vi "dotNET Crypto Demonstrator.vi"() -> ()   [LabVIEW 2021]
uses:
  Asymmetric Encryption/RSA/RSAEncryptionPadding.ctl
  Asymmetric Encryption/RSA/RSASignaturePadding.ctl
  Asymmetric Encryption/RSA/HashingAlgorithm.ctl
  Random Number Generation/dotNET Crypto RNG.lvlib
  Key Derivation/dotNET Crypto Key Derivation.lvlib
  Hashing/dotNET Crypto Hashing.lvlib
  Utility/dotNET Crypto Utility.lvlib
  Key Management/dotNET Crypto Key Management.lvlib
  Symmetric Encryption/dotNET Crypto Symmetric Encryption.lvlib
  System.Core
  Asymmetric Encryption/dotNET Crypto Asymmetric Encryption.lvlib
panel:
  in  "Tab Control":T1(tab)
  out "Random Data (hex string)":string
  in  "Gen RNG":bool
  out "Random Data (byte)":u8[](array[numeric])
  in  "# bytes":i32=32
  in  "Hashed Password (existing salt)":string
  out "Match?":bool
  in  "PBKDF2 Verify":bool
  in  "Salt":string
  in  "Hashed Password (random salt)":string
  in  "PBKDF2 Hash":bool
  in  "Password":string
  in  "HashingAlgorithm (SHA512)":T2=enum."SHA512"
  in  "Key length (64 bytes)":i32=64
  in  "saltSize (16 bytes)":i32=16
  in  "iterations (210000)":i32=210000
  in  "SHA512":bool
  in  "SHA384":bool
  in  "SHA256":bool
  in  "SHA1":bool
  in  "MD5":bool
  in  "Hash Out (hex string)":string
  in  "Data In":string
  in  "Hash Format":enum16{"ASCII", "Hex String"}(ring)
  in  "Cipher Block Mode":enum16{"ECB", "CBC"}(ring)=enum."CBC"
  in  "Initialisation Vector (hex string)":string
  in  "Create AES Key":bool
  in  "Key Size":enum16{"128 bit", "192 bit", "256 bit"}(ring)=enum."256 bit"
  in  "AES Key (hex string)":string
  in  "AES Encrypted Data":string
  in  "AES Raw Data":string
  in  "AES Encrypt":bool
  in  "AES Decrypt":bool
  in  "AES Encrypted Format":enum16{"ASCII", "Hex String"}(ring)=enum."Hex String"
  in  "AES Raw Format":enum16{"ASCII", "Hex String"}(ring)
  in  "Padding Mode":i32(ring)=3 items=["None"=1, "PKCS7"=2, "Zeros"=3, "ANSIX923"=4, "ISO10126"=5]
  in  "RSA Raw Format":enum16{"ASCII", "Hex String"}(ring)
  in  "RSA Encrypted Format":enum16{"ASCII", "Hex String"}(ring)=enum."Hex String"
  in  "RSA Decrypt":bool
  in  "RSA Encrypt":bool
  in  "Public Key (hex string)":string
  in  "Private Key (hex string)":string
  in  "Create RSA KeyPair":bool
  in  "RSA Encrypted Data":string
  in  "RSA Raw Data":string
  in  "keySize (2048 bit)":i32=2048
  in  "Padding Mode":T3=enum."OaepSHA512"
  out "Verified?":bool
  in  "RSASign Data Format":enum16{"ASCII", "Hex String"}(ring)
  in  "RSA Verify Data":bool
  in  "RSA Sign Data":bool
  in  "Signing Public Key (hex string)":string
  in  "Signing Private Key (hex string)":string
  in  "Create RSA Signing KeyPair":bool
  in  "Signature (hex string)":string
  in  "Data To Sign / Verify":string
  in  "keySize (2048 bit)":i32=2048
  in  "Signature Padding":T4
  in  "HashingAlgorithm":T2=enum."SHA512"
  in  "Key Length (bytes)":i32=64
  in  "Hash Algorithm":enum16{"HMACSHA256", "HMACSHA512"}(ring)
  in  "Generate Signature":bool
  in  "HMAC Signature (hex string)":string
  in  "HMAC Data Format":enum16{"ASCII", "Hex String"}(ring)
  in  "HMAC Data":string
  in  "HMAC Key (hex string)":string
  in  "Create HMAC Key":bool
  # ".NET Cryptography Library Playground"
  # "Generate random bytes of data using a cryptographically secure algorithm."
  # "Generates a fixed length key from an input password - can be used for key derivation or password hashing."
  # "Step 1: Generate a computationally intensive hash from the provided password."
  # "Step 2: Verify the password against the hash (reusing the previous salt above)"
  # "Generates a hash from the input data."
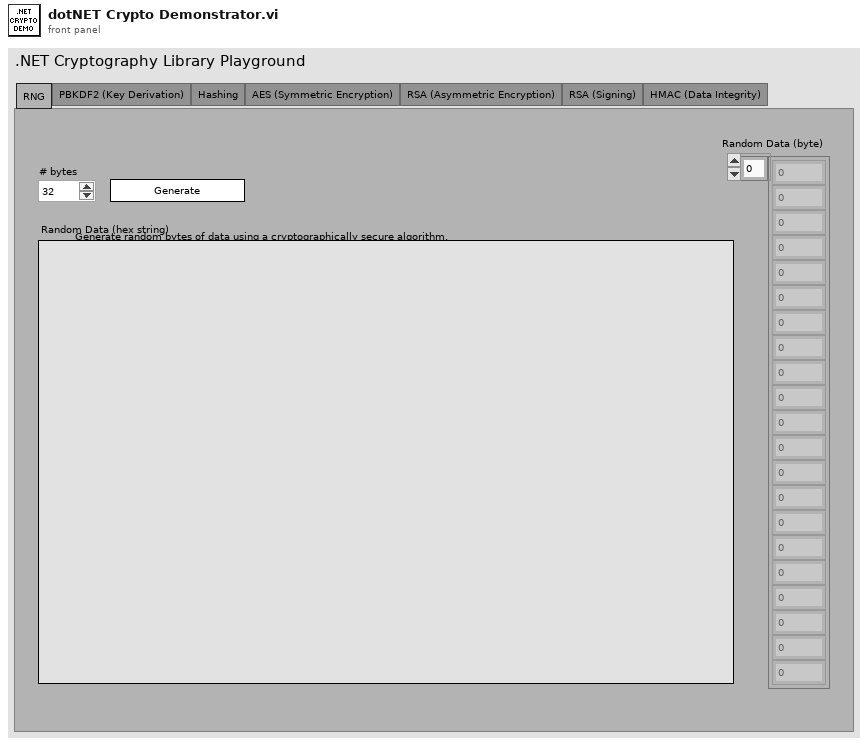
[diagram p1: front panel]
types:
  T1 = enum32{"RNG", "PBKDF2 (Key Derivation)", "Hashing", "AES (Symmetric Encryption)", "RSA (Asymmetric Encryption)", "RSA (Signing)", "HMAC (Data Integrity)"}
  T2 = typedef "dotNET Crypto Utility.lvlib/HashingAlgorithm.ctl" = enum16{"MD5", "SHA1", "SHA256", "SHA384", "SHA512"}
  T3 = typedef "dotNET Crypto Asymmetric Encryption.lvlib/RSAEncryptionPadding.ctl" = enum16{"OaepSHA1", "OaepSHA256", "OaepSHA384", "OaepSHA512", "Pkcs1"}
  T4 = typedef "dotNET Crypto Asymmetric Encryption.lvlib/RSASignaturePadding.ctl" = enum16{"Pkcs1", "Pss"}
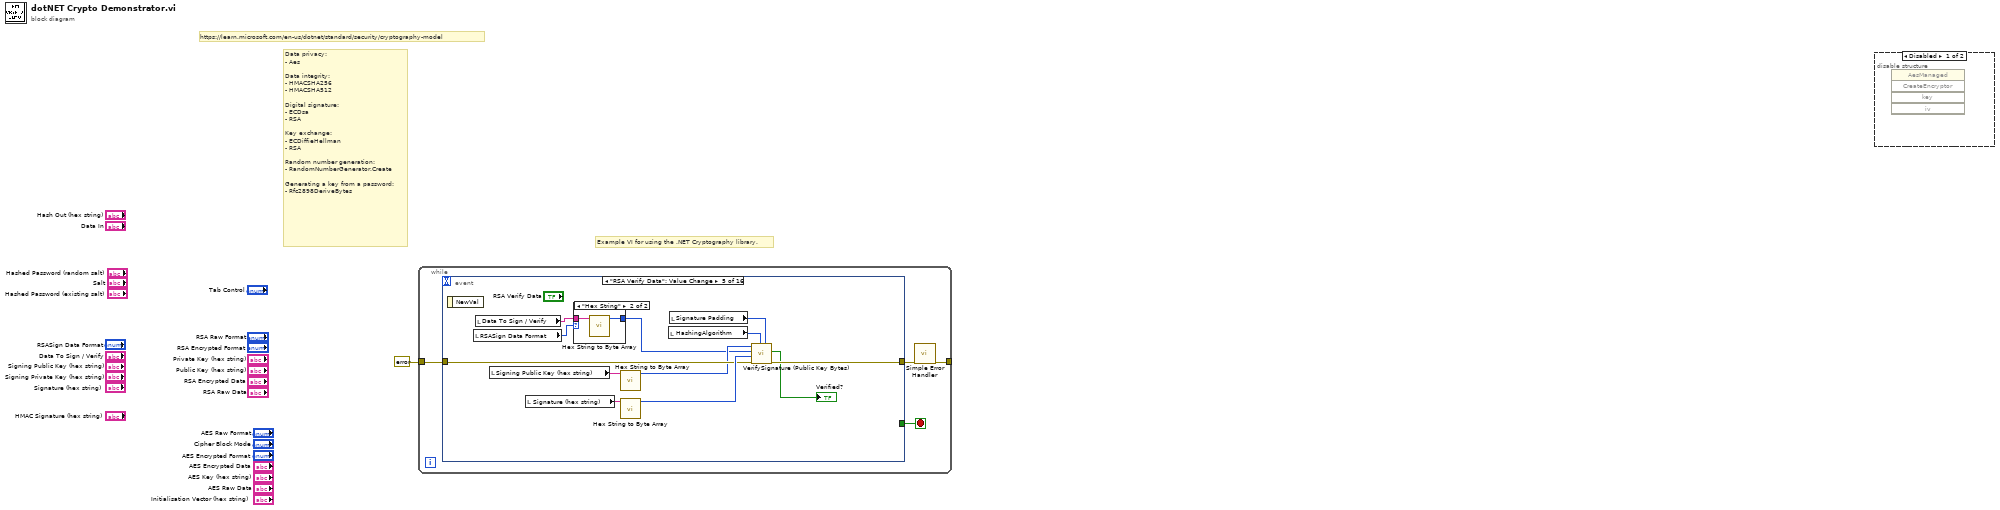
[diagram p0: block diagram]
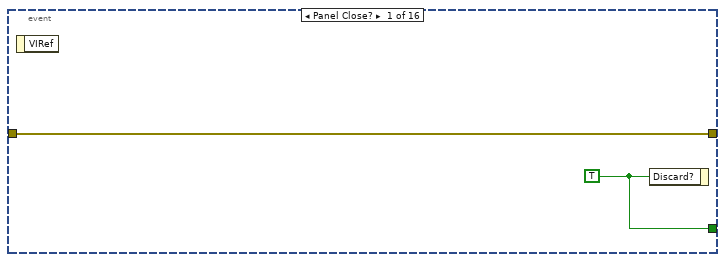
[diagram p2: hidden frame]
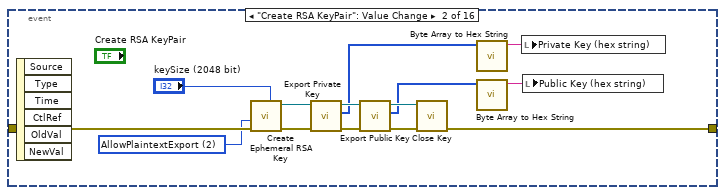
[diagram p3: hidden frame]
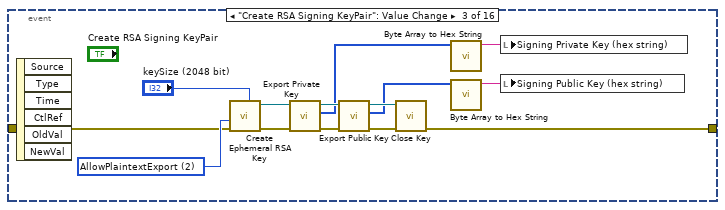
[diagram p4: hidden frame]
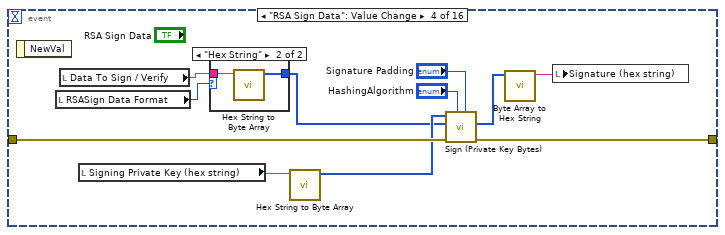
[diagram p5: hidden frame]
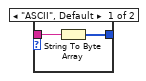
[diagram p6: hidden frame]
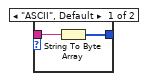
[diagram p7: hidden frame]
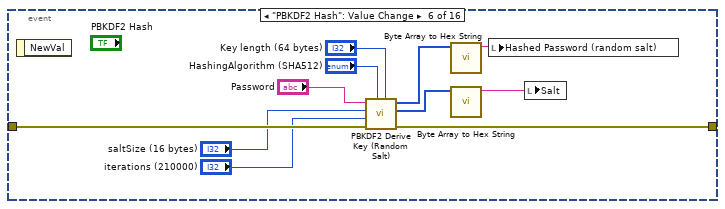
[diagram p8: hidden frame]
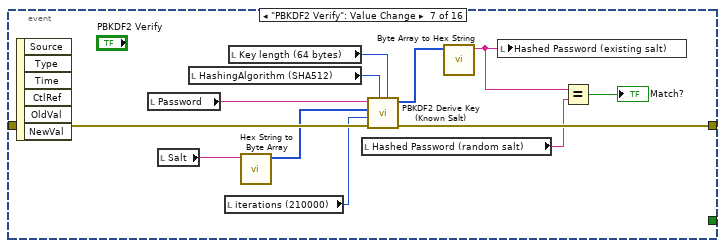
[diagram p9: hidden frame]
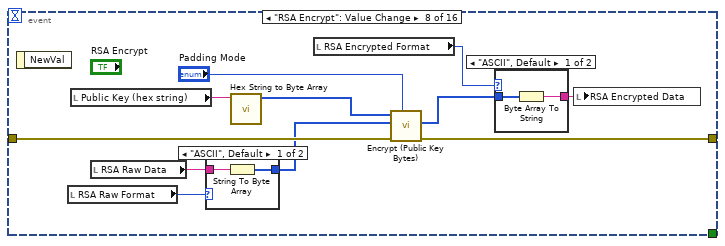
[diagram p10: hidden frame]
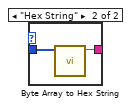
[diagram p11: hidden frame]
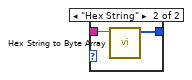
[diagram p12: hidden frame]
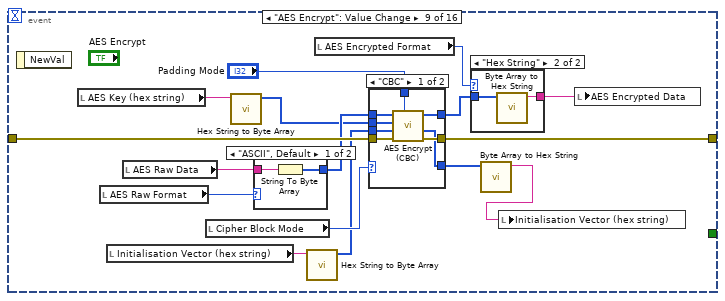
[diagram p13: hidden frame]
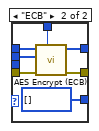
[diagram p14: hidden frame]
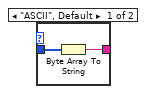
[diagram p15: hidden frame]
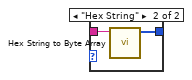
[diagram p16: hidden frame]
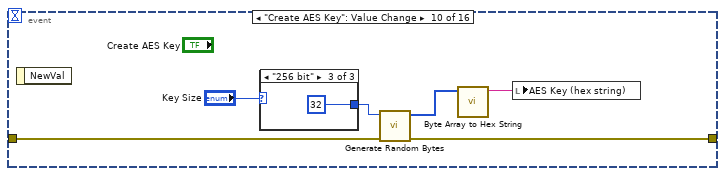
[diagram p17: hidden frame]
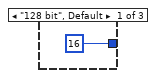
[diagram p18: hidden frame]
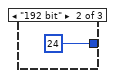
[diagram p19: hidden frame]
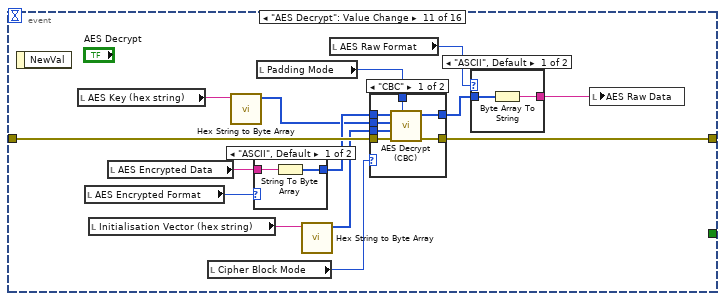
[diagram p20: hidden frame]
diagram:
  # "Example VI for using the .NET Cryptography library."
  # "https://learn.microsoft.com/en-us/dotnet/standard/security/cryptography-model"
  # "Data privacy:\n- Aes\n\nData integrity:\n- HMACSHA256\n- HMACSHA512\n\nDigital signature:\n- ECDsa\n- RSA\n\nKey exchange:\n- ECDiffieHellman\n- RSA\n\nRandom number generation:\n- RandomNumberGenerator.Create\n\nGenerating a key from a password:\n- Rfc2898DeriveBytes"
  n1 = while {
    tunnel: [w2] -> _
    tunnel: errorcluster {"status"=FALSE, "code"=0, "source"=""} ("error out") -> [w3]
    stop <- w5 stop-if-true
    n2 = event shown="[4] \"RSA Verify Data\": Value Change" {
      selector: _ -> [_ _ _ _ _ _ _ _ _ _ _ _ _ _ _ _]
      dyn-events: _ -> [_ _ _ _ _ _ _ _ _ _ _ _ _ _ _ _]
      timeout: _ -> [_ _ _ _ _ _ _ _ _ _ _ _ _ _ _ _]
      tunnel: [w7 _ _ _ _ _ _ _ _ _ _ _ _ _ _ _] -> w5
      tunnel: [w6 w17 w25 w46 w62 w76 w89 w93 w123 w150 w169 w195 w214 w223 w261 w280] -> w4
      tunnel: w3 -> [w6 w21 w26 w39 w53 w77 w88 w92 w124 w153 w170 w194 w213 w224 w262 w281]
      event Panel Close? {
        w7 = TRUE ("Discard?")
        n3 = event-data() -> ()  [unwired: 1 in, 1 out]
        n4 = event-data("Discard?"=w7) -> ()  [unwired: 1 in, 1 out]
      }
      event "Create RSA KeyPair": Value Change {
        w16 = 2 items=["None"=0, "AllowExport"=1, "AllowPlaintextExport"=2, "AllowArchiving"=4, "AllowPlaintextArchiving"=8] ("Export Policy (allow export)")
        n5 = event-data() -> ()  [unwired: 1 in, 6 out]
        n6 = call "Create Ephemeral RSA Key.vi"("Key Length (2048)"="keySize (2048 bit)", "error in (no error)"=w21, "Export Policy (allow export)"=w16) -> ("error out"=w15:errorcluster, "CngKey out"=w10:refnum<k24>)  [unwired: 7 in]
        n7 = call "Export Private Key.vi"("error in (no error)"=w15, "CngKey ref in"=w10) -> ("error out"=w14:errorcluster, "Private Key"=w9:u8[], "CngKey ref out"=w11:refnum<k24>)  [unwired: 7 in]
        n8 = call "Export Public Key.vi"("error in (no error)"=w14, "CngKey ref in"=w11) -> ("error out"=w13:errorcluster, "Public Key"=w8:u8[], "CngKey ref out"=w12:refnum<k24>)  [unwired: 7 in]
        n9 = call "Close Key.vi"("error in (no error)"=w13, "CngKey in"=w12) -> ("error out"=w17:errorcluster)  [unwired: 9 in]
        n10 = call "Byte Array to Hex String.vi"("Byte Array"=w9) -> ("Hex String"=w20:string)  [unwired: 10 in]
        n11 = call "Byte Array to Hex String.vi"("Byte Array"=w8) -> ("Hex String"=w19:string)  [unwired: 10 in]
        n12 = local write "Private Key (hex string)"(w20) -> ()
        n13 = local write "Public Key (hex string)"(w19) -> ()
      }
      event "Create RSA Signing KeyPair": Value Change {
        w33 = 2 items=["None"=0, "AllowExport"=1, "AllowPlaintextExport"=2, "AllowArchiving"=4, "AllowPlaintextArchiving"=8] ("Export Policy (allow export)")
        n14 = event-data() -> ()  [unwired: 1 in, 6 out]
        n15 = call "Create Ephemeral RSA Key.vi"("Key Length (2048)"="keySize (2048 bit)", "error in (no error)"=w26, "Export Policy (allow export)"=w33) -> ("error out"=w32:errorcluster, "CngKey out"=w27:refnum<k24>)  [unwired: 7 in]
        n16 = call "Export Private Key.vi"("error in (no error)"=w32, "CngKey ref in"=w27) -> ("error out"=w31:errorcluster, "Private Key"=w23:u8[], "CngKey ref out"=w28:refnum<k24>)  [unwired: 7 in]
        n17 = call "Export Public Key.vi"("error in (no error)"=w31, "CngKey ref in"=w28) -> ("error out"=w30:errorcluster, "Public Key"=w22:u8[], "CngKey ref out"=w29:refnum<k24>)  [unwired: 7 in]
        n18 = call "Close Key.vi"("error in (no error)"=w30, "CngKey in"=w29) -> ("error out"=w25:errorcluster)  [unwired: 9 in]
        n19 = call "Byte Array to Hex String.vi"("Byte Array"=w23) -> ("Hex String"=w35:string)  [unwired: 10 in]
        n20 = call "Byte Array to Hex String.vi"("Byte Array"=w22) -> ("Hex String"=w34:string)  [unwired: 10 in]
        n21 = local write "Signing Private Key (hex string)"(w35) -> ()
        n22 = local write "Signing Public Key (hex string)"(w34) -> ()
      }
      event "RSA Sign Data": Value Change {
        n23 = event-data() -> ()  [unwired: 1 in, 1 out]
        n24 = local read "RSASign Data Format"() -> (w43:enum16{"ASCII", "Hex String"})
        n25 = local read "Data To Sign / Verify"() -> (w42:string)
        n26 = local read "Signing Private Key (hex string)"() -> (w41:string)
        n27 = case shown="\"Hex String\"" w43 {
          tunnel: w42 -> [w48 w50]
          tunnel: [w47 w49] -> w36
          frame "ASCII", Default {
            n28 = String To Byte Array(string=w48) -> (unsigned byte array=w47:u8[])
          }
          frame "Hex String" {
            n29 = call "Hex String to Byte Array.vi"("Hex String"=w50) -> ("Byte Array"=w49:u8[])  [unwired: 10 in]
          }
        }
        n30 = call "Hex String to Byte Array.vi"("Hex String"=w41) -> ("Byte Array"=w37:u8[])  [unwired: 10 in]
        n31 = call "Sign (Private Key Bytes).vi"("RSASignPadding"="Signature Padding", "HashingAlgorithm"="HashingAlgorithm", "error in (no error)"=w39, "Data in"=w36, "Private key (bytes)"=w37) -> ("error out"=w46:errorcluster, "Signature out"=w38:u8[])  [unwired: 5 in]
        n32 = call "Byte Array to Hex String.vi"("Byte Array"=w38) -> ("Hex String"=w40:string)  [unwired: 10 in]
        n33 = local write "Signature (hex string)"(w40) -> ()
      }
      event "RSA Verify Data": Value Change {
        n34 = event-data() -> ()  [unwired: 1 in, 1 out]
        n35 = local read "RSASign Data Format"() -> (w61:enum16{"ASCII", "Hex String"})
        n36 = local read "Data To Sign / Verify"() -> (w60:string)
        n37 = local read "Signing Public Key (hex string)"() -> (w59:string)
        n38 = local read "Signature (hex string)"() -> (w56:string)
        n39 = case shown="\"Hex String\"" w61 {
          tunnel: w60 -> [w64 w66]
          tunnel: [w63 w65] -> w51
          frame "ASCII", Default {
            n40 = String To Byte Array(string=w64) -> (unsigned byte array=w63:u8[])
          }
          frame "Hex String" {
            n41 = call "Hex String to Byte Array.vi"("Hex String"=w66) -> ("Byte Array"=w65:u8[])  [unwired: 10 in]
          }
        }
        n42 = call "Hex String to Byte Array.vi"("Hex String"=w59) -> ("Byte Array"=w52:u8[])  [unwired: 10 in]
        n43 = call "Hex String to Byte Array.vi"("Hex String"=w56) -> ("Byte Array"=w55:u8[])  [unwired: 10 in]
        n44 = local read "HashingAlgorithm"() -> (w58:T2)
        n45 = local read "Signature Padding"() -> (w57:T4)
        n46 = call "VerifySignature (Public Key Bytes).vi"("RSASignPadding"=w57, "HashingAlgorithm"=w58, "error in (no error)"=w53, "Signature in"=w55, "Data in"=w51, "Public key in"=w52) -> ("error out"=w62:errorcluster, "Verified?"=→"Verified?":bool)  [unwired: 4 in]
      }
      event "PBKDF2 Hash": Value Change {
        n47 = event-data() -> ()  [unwired: 1 in, 1 out]
        n48 = call "PBKDF2 Derive Key (Random Salt).vi"("Key length (64 bytes)"="Key length (64 bytes)", "HashingAlgorithm (SHA512)"="HashingAlgorithm (SHA512)", "error in (no error)"=w77, "iterations (210000)"="iterations (210000)", "saltSize (16 bytes)"="saltSize (16 bytes)", "Password"="Password") -> ("error out"=w76:errorcluster, "Salt"=w69:u8[], "Derived Key"=w70:u8[])  [unwired: 3 in]
        n49 = call "Byte Array to Hex String.vi"("Byte Array"=w70) -> ("Hex String"=w68:string)  [unwired: 10 in]
        n50 = call "Byte Array to Hex String.vi"("Byte Array"=w69) -> ("Hex String"=w67:string)  [unwired: 10 in]
        n51 = local write "Hashed Password (random salt)"(w68) -> ()
        n52 = local write "Salt"(w67) -> ()
      }
      event "PBKDF2 Verify": Value Change {
        n53 = event-data() -> ()  [unwired: 1 in, 6 out]
        n54 = local read "Password"() -> (w82:string)
        n55 = local read "Salt"() -> (w83:string)
        n56 = local read "HashingAlgorithm (SHA512)"() -> (w85:T2)
        n57 = local read "iterations (210000)"() -> (w84:i32)
        n58 = local read "Key length (64 bytes)"() -> (w86:i32)
        n59 = call "Hex String to Byte Array.vi"("Hex String"=w83) -> ("Byte Array"=w87:u8[])  [unwired: 10 in]
        n60 = local read "Hashed Password (random salt)"() -> (w78:string)
        n61 = call "PBKDF2 Derive Key (Known Salt).vi"("Key length (64 bytes)"=w86, "HashingAlgorithm (SHA512)"=w85, "error in (no error)"=w88, "iterations (210000)"=w84, "Salt"=w87, "Password"=w82) -> ("error out"=w89:errorcluster, "Derived Key"=w81:u8[])  [unwired: 4 in]
        n62 = call "Byte Array to Hex String.vi"("Byte Array"=w81) -> ("Hex String"=w79:string)  [unwired: 10 in]
        n63 = local write "Hashed Password (existing salt)"(w79) -> ()
        n64 = Equal?(x=w79, y=w78) -> (x = y?=→"Match?":bool)
      }
      event "RSA Encrypt": Value Change {
        n65 = event-data() -> ()  [unwired: 1 in, 1 out]
        n66 = local read "RSA Raw Format"() -> (w96:enum16{"ASCII", "Hex String"})
        n67 = local read "Public Key (hex string)"() -> (w99:string)
        n68 = local read "RSA Raw Data"() -> (w98:string)
        n69 = case shown="\"ASCII\", Default" w96 {
          tunnel: w98 -> [w106 w108]
          tunnel: [w105 w107] -> w90
          frame "ASCII", Default {
            n70 = String To Byte Array(string=w106) -> (unsigned byte array=w105:u8[])
          }
          frame "Hex String" {
            n71 = call "Hex String to Byte Array.vi"("Hex String"=w108) -> ("Byte Array"=w107:u8[])  [unwired: 10 in]
          }
        }
        n72 = call "Hex String to Byte Array.vi"("Hex String"=w99) -> ("Byte Array"=w91:u8[])  [unwired: 10 in]
        n73 = local read "RSA Encrypted Format"() -> (w95:enum16{"ASCII", "Hex String"})
        n74 = call "Encrypt (Public Key Bytes).vi"("Padding Mode"="Padding Mode", "error in (no error)"=w92, "Raw data in"=w90, "Public key in"=w91) -> ("error out"=w93:errorcluster, "Encrypted data out"=w94:u8[])  [unwired: 6 in]
        n75 = case shown="\"ASCII\", Default" w95 {
          tunnel: w94 -> [w102 w104]
          tunnel: [w101 w103] -> w97
          frame "ASCII", Default {
            n76 = Byte Array To String(unsigned byte array=w102) -> (string=w101:string)
          }
          frame "Hex String" {
            n77 = call "Byte Array to Hex String.vi"("Byte Array"=w104) -> ("Hex String"=w103:string)  [unwired: 10 in]
          }
        }
        n78 = local write "RSA Encrypted Data"(w97) -> ()
      }
      event "AES Encrypt": Value Change {
        n79 = event-data() -> ()  [unwired: 1 in, 1 out]
        n80 = local read "AES Key (hex string)"() -> (w122:string)
        n81 = local read "AES Raw Format"() -> (w117:enum16{"ASCII", "Hex String"})
        n82 = local read "Initialisation Vector (hex string)"() -> (w110:string)
        n83 = local read "AES Raw Data"() -> (w121:string)
        n84 = local read "Cipher Block Mode"() -> (w113:enum16{"ECB", "CBC"})
        n85 = call "Hex String to Byte Array.vi"("Hex String"=w122) -> ("Byte Array"=w115:u8[])  [unwired: 10 in]
        n86 = case shown="\"ASCII\", Default" w117 {
          tunnel: w121 -> [w145 w147]
          tunnel: [w144 w146] -> w120
          frame "ASCII", Default {
            n87 = String To Byte Array(string=w145) -> (unsigned byte array=w144:u8[])
          }
          frame "Hex String" {
            n88 = call "Hex String to Byte Array.vi"("Hex String"=w147) -> ("Byte Array"=w146:u8[])  [unwired: 10 in]
          }
        }
        n89 = call "Hex String to Byte Array.vi"("Hex String"=w110) -> ("Byte Array"=w109:u8[])  [unwired: 10 in]
        n90 = local read "AES Encrypted Format"() -> (w116:enum16{"ASCII", "Hex String"})
        n91 = case shown="\"CBC\"" w113 {
          tunnel: w124 -> [w132 w139]
          tunnel: [w131 w138] -> w123
          tunnel: w120 -> [w129 w137]
          tunnel: [w130 w136] -> w119
          tunnel: w115 -> [w128 w135]
          tunnel: "Padding Mode" -> [w127 w134]
          tunnel: [w126 u8[] [] ("IV out")] -> w112
          tunnel: w109 -> [w125 _]
          frame "CBC" {
            n92 = call "AES Encrypt (CBC).vi"("Padding"=w127, "error in (no error)"=w132, "IV"=w125, "Key"=w128, "Raw data in"=w129) -> ("error out"=w131:errorcluster, "IV out"=w126:u8[], "Encrypted data out"=w130:u8[])  [unwired: 4 in]
          }
          frame "ECB" {
            n93 = call "AES Encrypt (ECB).vi"("Padding"=w134, "error in (no error)"=w139, "Key"=w135, "Raw data in"=w137) -> ("error out"=w138:errorcluster, "Encrypted data out"=w136:u8[])  [unwired: 6 in]
          }
        }
        n94 = case shown="\"Hex String\"" w116 {
          tunnel: w119 -> [w141 w143]
          tunnel: [w140 w142] -> w118
          frame "ASCII", Default {
            n95 = Byte Array To String(unsigned byte array=w141) -> (string=w140:string)
          }
          frame "Hex String" {
            n96 = call "Byte Array to Hex String.vi"("Byte Array"=w143) -> ("Hex String"=w142:string)  [unwired: 10 in]
          }
        }
        n97 = call "Byte Array to Hex String.vi"("Byte Array"=w112) -> ("Hex String"=w111:string)  [unwired: 10 in]
        n98 = local write "Initialisation Vector (hex string)"(w111) -> ()
        n99 = local write "AES Encrypted Data"(w118) -> ()
      }
      event "Create AES Key": Value Change {
        n100 = event-data() -> ()  [unwired: 1 in, 1 out]
        n101 = case shown="\"256 bit\"" "Key Size" {
          tunnel: [16 24 32] -> w148
          frame "128 bit", Default {
          }
          frame "192 bit" {
          }
          frame "256 bit" {
          }
        }
        n102 = call "Generate Random Bytes.vi"("error in (no error)"=w153, "byte count"=w148) -> ("error out"=w150:errorcluster, "random data (U8)"=w152:u8[])  [unwired: 8 in]
        n103 = call "Byte Array to Hex String.vi"("Byte Array"=w152) -> ("Hex String"=w151:string)  [unwired: 10 in]
        n104 = local write "AES Key (hex string)"(w151) -> ()
      }
      event "AES Decrypt": Value Change {
        n105 = event-data() -> ()  [unwired: 1 in, 1 out]
        n106 = local read "AES Key (hex string)"() -> (w168:string)
        n107 = local read "AES Encrypted Format"() -> (w163:enum16{"ASCII", "Hex String"})
        n108 = local read "Initialisation Vector (hex string)"() -> (w159:string)
        n109 = local read "AES Encrypted Data"() -> (w167:string)
        n110 = local read "Cipher Block Mode"() -> (w158:enum16{"ECB", "CBC"})
        n111 = call "Hex String to Byte Array.vi"("Hex String"=w168) -> ("Byte Array"=w161:u8[])  [unwired: 10 in]
        n112 = case shown="\"ASCII\", Default" w163 {
          tunnel: w167 -> [w189 w191]
          tunnel: [w188 w190] -> w166
          frame "ASCII", Default {
            n113 = String To Byte Array(string=w189) -> (unsigned byte array=w188:u8[])
          }
          frame "Hex String" {
            n114 = call "Hex String to Byte Array.vi"("Hex String"=w191) -> ("Byte Array"=w190:u8[])  [unwired: 10 in]
          }
        }
        n115 = local read "Padding Mode"() -> (w160:i32)
        n116 = call "Hex String to Byte Array.vi"("Hex String"=w159) -> ("Byte Array"=w157:u8[])  [unwired: 10 in]
        n117 = local read "AES Raw Format"() -> (w162:enum16{"ASCII", "Hex String"})
        n118 = case shown="\"CBC\"" w158 {
          tunnel: w170 -> [w176 w183]
          tunnel: [w175 w182] -> w169
          tunnel: w166 -> [w177 w181]
          tunnel: [w174 w180] -> w165
          tunnel: w161 -> [w172 w179]
          tunnel: w160 -> [w173 w178]
          tunnel: w157 -> [w171 _]
          frame "CBC" {
            n119 = call "AES Decrypt (CBC).vi"("Padding"=w173, "error in (no error)"=w176, "IV"=w171, "Key"=w172, "Encrypted data in"=w177) -> ("error out"=w175:errorcluster, "Raw data out"=w174:u8[])  [unwired: 5 in]
          }
          frame "ECB" {
            n120 = call "AES Decrypt (ECB).vi"("Padding"=w178, "error in (no error)"=w183, "Key"=w179, "Encrypted data in"=w181) -> ("error out"=w182:errorcluster, "Raw data out"=w180:u8[])  [unwired: 6 in]
          }
        }
        n121 = case shown="\"ASCII\", Default" w162 {
          tunnel: w165 -> [w185 w187]
          tunnel: [w184 w186] -> w164
          frame "ASCII", Default {
            n122 = Byte Array To String(unsigned byte array=w185) -> (string=w184:string)
          }
          frame "Hex String" {
            n123 = call "Byte Array to Hex String.vi"("Byte Array"=w187) -> ("Hex String"=w186:string)  [unwired: 10 in]
          }
        }
        n124 = local write "AES Raw Data"(w164) -> ()
      }
      event "RSA Decrypt": Value Change {
        n125 = event-data() -> ()  [unwired: 1 in, 1 out]
        n126 = local read "RSA Encrypted Format"() -> (w197:enum16{"ASCII", "Hex String"})
        n127 = local read "RSA Encrypted Data"() -> (w201:string)
        n128 = local read "Private Key (hex string)"() -> (w202:string)
        n129 = case shown="\"Hex String\"" w197 {
          tunnel: w201 -> [w204 w206]
          tunnel: [w203 w205] -> w192
          frame "ASCII", Default {
            n130 = String To Byte Array(string=w204) -> (unsigned byte array=w203:u8[])
          }
          frame "Hex String" {
            n131 = call "Hex String to Byte Array.vi"("Hex String"=w206) -> ("Byte Array"=w205:u8[])  [unwired: 10 in]
          }
        }
        n132 = call "Hex String to Byte Array.vi"("Hex String"=w202) -> ("Byte Array"=w193:u8[])  [unwired: 10 in]
        n133 = local read "Padding Mode"() -> (w199:T3)
        n134 = local read "RSA Raw Format"() -> (w198:enum16{"ASCII", "Hex String"})
        n135 = call "Decrypt (Private Key Bytes).vi"("Padding Mode"=w199, "error in (no error)"=w194, "Encrypted data in"=w192, "Private key in"=w193) -> ("error out"=w195:errorcluster, "Raw data out"=w196:u8[])  [unwired: 6 in]
        n136 = case shown="\"ASCII\", Default" w198 {
          tunnel: w196 -> [w208 w210]
          tunnel: [w207 w209] -> w200
          frame "ASCII", Default {
            n137 = Byte Array To String(unsigned byte array=w208) -> (string=w207:string)
          }
          frame "Hex String" {
            n138 = call "Byte Array to Hex String.vi"("Byte Array"=w210) -> ("Hex String"=w209:string)  [unwired: 10 in]
          }
        }
        n139 = local write "RSA Raw Data"(w200) -> ()
      }
      event "Gen RNG": Value Change {
        n140 = event-data() -> ()  [unwired: 1 in, 1 out]
        n141 = call "Generate Random Bytes.vi"("error in (no error)"=w213, "byte count"="# bytes") -> ("error out"=w214:errorcluster, "random data (U8)"=w212:u8[])  [unwired: 8 in]
        "Random Data (byte)" <- w212
        n142 = call "Byte Array to Hex String.vi"("Byte Array"=w212) -> ("Hex String"=→"Random Data (hex string)":string)  [unwired: 10 in]
      }
      event "MD5", "SHA1", "SHA256", "SHA384", "SHA512": Value Change {
        n143 = event-data() -> ("CtlRef"=w217:refnum<vi>)  [unwired: 1 in]
        n144 = property class="Bool"(reference=w217) -> ("Label.Text"=w216:string)  [unwired: 1 in, 2 out]
        n145 = local read "Data In"() -> (w222:string)
        n146 = case shown="\"Hex String\"" "Hash Format" {
          tunnel: w222 -> [w250 w252]
          tunnel: [w249 w251] -> w220
          frame "Hex String" {
            n147 = call "Hex String to Byte Array.vi"("Hex String"=w250) -> ("Byte Array"=w249:u8[])  [unwired: 10 in]
          }
          frame "ASCII" {
            n148 = String To Byte Array(string=w252) -> (unsigned byte array=w251:u8[])
          }
        }
        n149 = case shown="Default" w216 {
          tunnel: w224 -> [w228 w231 w236 w240 w244 w248]
          tunnel: [w226 w230 w233 w237 w242 w247] -> w223
          tunnel: [u8[] [] ("MD5 Hash") w229 w234 w238 w241 w246] -> w221
          tunnel: w220 -> [_ w232 w235 w239 w243 w245]
          frame Default {
            n150 = call <vilib>:"Error Cluster From Error Code.vi"("error in (no error)"=w228, "error code (0)"=1) -> ("error out"=w226:errorcluster)  [unwired: 7 in]
          }
          frame "sha1" {
            n151 = call "SHA1.vi"("error in (no error)"=w231, "Data in"=w232) -> ("error out"=w230:errorcluster, "SHA1 Hash"=w229:u8[])  [unwired: 8 in]
          }
          frame "sha256" {
            n152 = call "SHA256.vi"("error in (no error)"=w236, "Data in"=w235) -> ("error out"=w233:errorcluster, "SHA256 Hash"=w234:u8[])  [unwired: 8 in]
          }
          frame "sha384" {
            n153 = call "SHA384.vi"("error in (no error)"=w240, "Data in"=w239) -> ("error out"=w237:errorcluster, "SHA384 Hash"=w238:u8[])  [unwired: 8 in]
          }
          frame "sha512" {
            n154 = call "SHA512.vi"("error in (no error)"=w244, "Data in"=w243) -> ("error out"=w242:errorcluster, "SHA512 Hash"=w241:u8[])  [unwired: 8 in]
          }
          frame "md5" {
            n155 = call "MD5.vi"("error in (no error)"=w248, "Data in"=w245) -> ("error out"=w247:errorcluster, "MD5 Hash"=w246:u8[])  [unwired: 8 in]
          }
        }
        n156 = call "Byte Array to Hex String.vi"("Byte Array"=w221) -> ("Hex String"=w219:string)  [unwired: 10 in]
        n157 = local write "Hash Out (hex string)"(w219) -> ()
      }
      event "Generate Signature": Value Change {
        n158 = event-data() -> ()  [unwired: 1 in, 1 out]
        n159 = case shown="\"ASCII\", Default" "HMAC Data Format" {
          tunnel: "HMAC Data" -> [w274 w276]
          tunnel: [w273 w275] -> w254
          frame "ASCII", Default {
            n160 = String To Byte Array(string=w274) -> (unsigned byte array=w273:u8[])
          }
          frame "Hex String" {
            n161 = call "Hex String to Byte Array.vi"("Hex String"=w276) -> ("Byte Array"=w275:u8[])  [unwired: 10 in]
          }
        }
        n162 = call "Hex String to Byte Array.vi"("Hex String"="HMAC Key (hex string)") -> ("Byte Array"=w259:u8[])  [unwired: 10 in]
        n163 = case shown="\"HMACSHA256\"" "Hash Algorithm" {
          tunnel: w262 -> [w267 w272]
          tunnel: [w263 w271] -> w261
          tunnel: w259 -> [w265 w270]
          tunnel: [w264 w269] -> w258
          tunnel: w254 -> [w266 w268]
          frame "HMACSHA512" {
            n164 = call "HMACSHA512.vi"("error in (no error)"=w267, "Key in"=w265, "Data in"=w266) -> ("error out"=w263:errorcluster, "HMACSHA512 Hash"=w264:u8[])  [unwired: 7 in]
          }
          frame "HMACSHA256" {
            n165 = call "HMACSHA256.vi"("error in (no error)"=w272, "Key in"=w270, "Data in"=w268) -> ("error out"=w271:errorcluster, "HMACSHA256 Hash"=w269:u8[])  [unwired: 7 in]
          }
        }
        n166 = call "Byte Array to Hex String.vi"("Byte Array"=w258) -> ("Hex String"=w257:string)  [unwired: 10 in]
        n167 = local write "HMAC Signature (hex string)"(w257) -> ()
      }
      event "Create HMAC Key": Value Change {
        n168 = event-data() -> ()  [unwired: 1 in, 6 out]
        n169 = call "Generate Random Bytes.vi"("error in (no error)"=w281, "byte count"="Key Length (bytes)") -> ("error out"=w280:errorcluster, "random data (U8)"=w279:u8[])  [unwired: 8 in]
        n170 = call "Byte Array to Hex String.vi"("Byte Array"=w279) -> ("Hex String"=w278:string)  [unwired: 10 in]
        n171 = local write "HMAC Key (hex string)"(w278) -> ()
      }
    }
    n172 = call <vilib>:"Simple Error Handler.vi"("error in (no error)"=w4) -> ("error out"=w2:errorcluster)  [unwired: 4 in, 4 out]
  }
  n173 = disable-structure shown="Disabled" {
    frame Disabled {
      n174 = invoke class="AesManaged" method="CreateEncryptor"() -> ()  [unwired: 5 in, 5 out]
    }
    frame Enabled {
    }
  }
